vi "From Variant.vi"(8 "error in (no error)":errorcluster, 11 "Variant":variant) -> (0 "error out":errorcluster, 3 "Assertion out":refnum<class "Assertion.lvclass">)   [LabVIEW 2017, in "Assertion.lvclass"]
uses:
  <vilib>/gpm_packages/@cs/data-type-serializer/source/Assertion/Assertion.lvclass
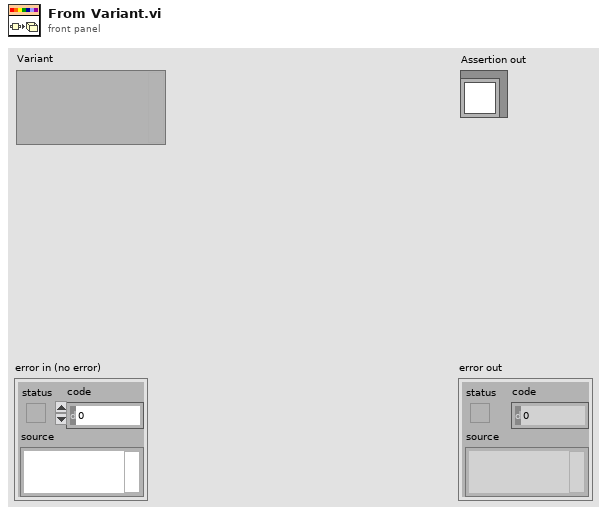
[diagram p1: front panel]
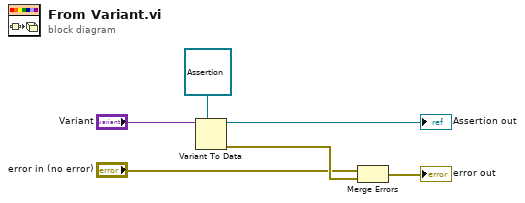
[diagram p0: block diagram]
diagram:
  n1 = Variant To Data(type=refnum<class "Assertion.lvclass"> refnum ("Boolean in"), Variant="Variant") -> (data=→"Assertion out":refnum<class "Assertion.lvclass">, error out=w5:errorcluster)  [unwired: 1 in]
  n2 = Merge Errors("error in (no error)", w5) -> (→"error out":errorcluster)
